vi "RT Driver VI.vi"(7 "Operation":T1, 11 "Device Reference in":T2 format="%.0x") -> (0 "Error Code":i32)   [LabVIEW 2023, in "Protection and Counter Addon Engine.lvlib"]
uses:
  Protection and Counter Addon Engine.lvlib
  <vilib>/NI VeriStand/Custom Device API/Custom Device Item Ref.ctl
  <vilib>/NI VeriStand/Custom Device API/Hardware Interface Driver VI Operation.ctl
  <vilib>/NI/NIVS Inline Async API/_VS Inline Async API/VS Inline Async API/Types/Error Handling Settings.ctl
  Addon Shared/Types/Exported.OnCompile.ctl
  Addon Shared/Types/XNET Settings.ctl
  SubModules/Frame-Protection-Support/Source/Shared/Types/Exported Frame Settings.ctl
  SubModules/Frame-Protection-Support/Source/Shared/Types/Exported Frame Type.ctl
  SubModules/Frame-Protection-Support/Source/Shared/Types/Exported Protection Settings.ctl
  SubModules/Frame-Protection-Support/Source/Shared/Types/Protection Type.ctl
  SubModules/Frame-Protection-Support/Source/Shared/Types/XNET Signal Configuration.ctl
  SubModules/Frame-Protection-Support/Source/Shared/Types/Exported Counter Settings.ctl
  SubModules/Frame-Protection-Support/Source/Shared/Types/Exported Event Trigger Type.ctl
  Addon Shared/Types/986x.ctl
  <vilib>/NI/NIVS Inline Async API/_VS Inline Async API/VS Inline Async API/VS Inline Async API.lvclass
  Types/RT Async Engine Settings.ctl
  SubModules/Frame-Protection-Support/Source/Engine/Types/RT Frame Settings.ctl
  SubModules/Frame-Protection-Support/Source/Engine/Types/RT Protection Configuration.ctl
  SubModules/Frame-Protection-Support/Source/Engine/Types/RT Frame Incoming Values.ctl
  <vilib>/NI/NIVS Inline Async API/_VS Inline Async API/VS Inline Async API/VS Inline Async API.lvclass/VS Inline Async API.ctl
  <vilib>/NI/NIVS Inline Async API/_Data Access Engine/Data Access Engine/Data Access Engine.lvclass/Data Access Engine.ctl
  <vilib>/NI/NIVS Inline Async API/_Data Access Engine/Access Type Classes/Write/Write.lvclass/Write.ctl
  <vilib>/NI/NIVS Inline Async API/_Data Access Engine/Access Type Classes/ReadWrite/ReadWrite.lvclass/ReadWrite.ctl
  <vilib>/NI/NIVS Inline Async API/_Data Access Engine/Access Type Classes/Read/Read.lvclass/Read.ctl
  SubVIs/Bitfile.Initialize.vi
  SubModules/Frame-Protection-Support/Source/Engine/SubVIs/Initialize Protection Frames Outgoing.vi
  <vilib>/NI/NIVS Inline Async API/_Data Access Engine/Data Access Engine/Methods/Data.Engine.Read Data from HW.vi
  <vilib>/NI/NIVS Inline Async API/_VS Inline Async API/Error Handling Process/SubVIs/Error.GetError.vi
  <vilib>/NI/NIVS Inline Async API/_Data Access Engine/Data Access Engine/Methods/Data.Engine.Write Data to HW.vi
  SubVIs/Bitfile.Download.vi
  <vilib>/NI/NIVS Inline Async API/_Data Access Engine/Access Type Classes/ReadWrite/ReadWrite.EngineData.vi
  <vilib>/NI/NIVS Inline Async API/_Data Access Engine/Access Type Classes/Write/Write.EngineData.vi
  <vilib>/NI/NIVS Inline Async API/_Data Access Engine/Access Type Classes/Read/Read.EngineData.vi
  <vilib>/NI VeriStand/Custom Device API/NI VeriStand - Get Channel Value by Data Reference.vi
  <vilib>/NI VeriStand/Custom Device API/NI VeriStand - Set Channel Value by Data Reference.vi
  <vilib>/NI VeriStand/Custom Device API/NI VeriStand - Get Channel Values by Block Data Reference.vi
  Addon Shared/SubVIs/GUID Lookup.vi
  <vilib>/NI VeriStand/Custom Device API/Get Item Property (Variant).vi
  <vilib>/Utility/libraryn.llb/Check if File or Folder Exists.vi
  <vilib>/Utility/error.llb/Error Cluster From Error Code.vi
  <vilib>/rvi/Utilities/XML/nirviXML_GetValue.vi
  <vilib>/rvi/Utilities/XML/nirviXML_GetValue_String.vi
  <vilib>/xnet/xnet.llb/XNET Create Session.vi
  <vilib>/xnet/xnet.llb/XNET Create Session (Frame Output Stream).vi
  <vilib>/xnet/xnet.llb/XNET Create Session (Conversion).vi
  SubModules/Frame-Protection-Support/Source/LP_CRC/Re-order Protection Configs.vi
  SubModules/Frame-Protection-Support/Source/Engine/SubVIs/Initialize Protection Frames Incoming.vi
  <vilib>/xnet/xnet.llb/XNET Create Session (Frame Input Stream).vi
  <vilib>/Utility/SystemLogging/Write to System Log.vi
  <vilib>/NI VeriStand/Custom Device API/Global Data Refs.vi
  <vilib>/NI VeriStand/Custom Device API/Custom Device API.lvlib
  Addon Shared/Protection and Counter Addon Shared.lvlib
  SubModules/Frame-Protection-Support/Source/Shared/Protection and Counter Support Shared.lvlib
  <vilib>/NI VeriStand/Custom Device Tools/Custom Device Utility Library/Custom Device Utility Library.lvlib
  SubModules/Frame-Protection-Support/Source/Engine/Protection and Counter Support Engine.lvlib
  SubModules/Frame-Protection-Support/Source/LP_CRC/LP_CRC.lvlib
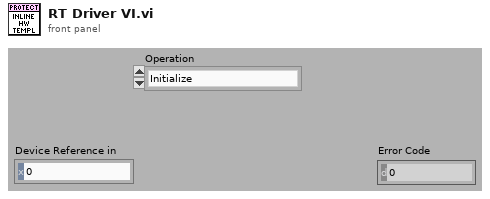
[diagram p1: front panel]
types:
  T1 = typedef "Custom Device API.lvlib/Hardware Interface Driver VI Operation.ctl" = enum16{"Initialize", "Start", "Read Data from HW", "Write Data to HW", "Close"}
  T2 = typedef "Custom Device API.lvlib/Custom Device Item Ref.ctl" = u64
  T3 = typedef "Protection and Counter Addon Engine.lvlib/RT Async Engine Settings.ctl" = cluster{"Name":string, "Priority":i32, "XNET Settings":T4, "FPGA Session":u32, "Outgoing CAN Session":refnum<k21>, "Outgoing Frame Count":i32, "Outgoing Frames":T5[], "Incoming CAN Session":refnum<k21>, "Incoming Frame Count":i32, "Incoming Frames":T5[], "Incoming Values":T12}
  T4 = typedef "Protection and Counter Addon Shared.lvlib/XNET Settings.ctl" = cluster{"Database":refnum<k21>, "Cluster":refnum<k21>, "Port":string, "Baud rate [Bd]":u64, "Termination":u32, "CAN I/O Mode":u32, "FD Baud rate [Bd]":u64, "Priority":i32, "Use Legacy":bool, "FD ISO Mode":u32}
  T5 = typedef "Protection and Counter Support Engine.lvlib/RT Frame Settings.ctl" = cluster{"Type":T6, "Frame ID":u32, "Payload Length":u32, "VS Offset":i32, "VS Length":i32, "Frame Conversion":refnum<k21>, "Frame.Data":dbl[], "Generation Period":u32, "Time Since Last Generation":u32, "Generation Iterations":u32, "Generation Counter":u32, "Has Protection?":bool, "Protection Configurations":T7[], "Has Counter?":bool, "Counter Configurations":T10[], "Has Disable?":bool, "Disable VS Index":i32, "Transmit Trigger":T11, "Trigger VS Index":i32}
  T6 = typedef "Protection and Counter Support Shared.lvlib/Exported Frame Type.ctl" = enum16{"Periodic", "Event", "Periodic/Event"}
  T7 = typedef "Protection and Counter Support Engine.lvlib/RT Protection Configuration.ctl" = cluster{"Protection Frame Index":i32, "Protection Type":T8, "Data Indeces":i32[], "Data Array":dbl[], "Check Sum Conversion":refnum<k21>, "CRC Channels":T9[], "Protection VS Index":i32, "Counter Data Index":i32, "Override Index":i32, "Override Value Index":i32, "Map":map{i32, u8[]}}
  T8 = typedef "Protection and Counter Support Shared.lvlib/Protection Type.ctl" = enum16{"Arb ID + Bytes Checksum with Inversion", "Arb ID + Bytes CRC with Inversion", "Reversed Raw Signal Checksum with Inversion", "Concatenated Two's Compliment", "LP_CRC8", "LP_Checksum", "LP_CRC8_MRS"}
  T9 = typedef "Protection and Counter Support Shared.lvlib/XNET Signal Configuration.ctl" = cluster{"Start Bit":i32, "Name":string, "Number of bits":i32, "Scale":dbl, "Offset":dbl, "Data Type":u32, "Counter":bool}
  T10 = typedef "Protection and Counter Support Shared.lvlib/Exported Counter Settings.ctl" = cluster{"Frame Index":i32, "Max Count":dbl, "VS Index":i32, "Bit Length":i64, "Override Index":i32, "Override Value Index":i32}
  T11 = typedef "Protection and Counter Support Shared.lvlib/Exported Event Trigger Type.ctl" = enum16{"Channel value change", "Trigger channel (not zero)", "Channel value change or trigger channel (not zero)", "Trigger channel (any value change)", "Channel value change or trigger channel (any value change)"}
  T12 = typedef "Protection and Counter Support Engine.lvlib/RT Frame Incoming Values.ctl" = cluster{"Signal Values":dbl[], "Signal Invalid Values":dbl[], "ProtCtr Sig Values":dbl[], "Timestamps":timestamp[], "Time Differences":dbl[], "IDs":u32[]}
  T13 = cluster{"Process":refnum<class "VS Inline Async API.lvclass">, "RT Configuration":T3}
  T14 = typedef "VS Inline Async API.lvlib/VS Inline Async API.lvclass/Error Handling Settings.ctl" = cluster{"Write to SystemLog (F)":bool}
  T15 = typedef "Protection and Counter Addon Shared.lvlib/Exported.OnCompile.ctl" = cluster{"Name":string, "XNET Settings":T4, "Frames":T16[], "986x Support":T18, "Incoming Frames":T16[]}
  T16 = typedef "Protection and Counter Support Shared.lvlib/Exported Frame Settings.ctl" = cluster{"Type":T6, "Frame ID":u32, "Payload Length":u32, "Signal XNET Paths":string[], "Frame.PrevData":dbl[], "VS Offset":i32, "VS Length":i32, "Generation Period":u32, "Has Protection?":bool, "Protection Configurations":T17[], "Has Counter":bool, "Counter Configurations":T10[], "Has Disable?":bool, "Disable VS Index":i32, "Transmit Trigger":T11, "Trigger VS Index":i32}
  T17 = typedef "Protection and Counter Support Shared.lvlib/Exported Protection Settings.ctl" = cluster{"Protection Frame Index":i32, "Protection Type":T8, "Data Indeces":i32[], "Initialized Data Array":dbl[], "Protection Signal XNET Paths":string[], "CRC Channels":T9[], "Protection VS Update Index":i32, "Override Index":i32, "Override Value Index":i32}
  T18 = typedef "Protection and Counter Addon Shared.lvlib/986x.ctl" = cluster{"Enable":bool, "RIO Device":string, "Bitfile":path}
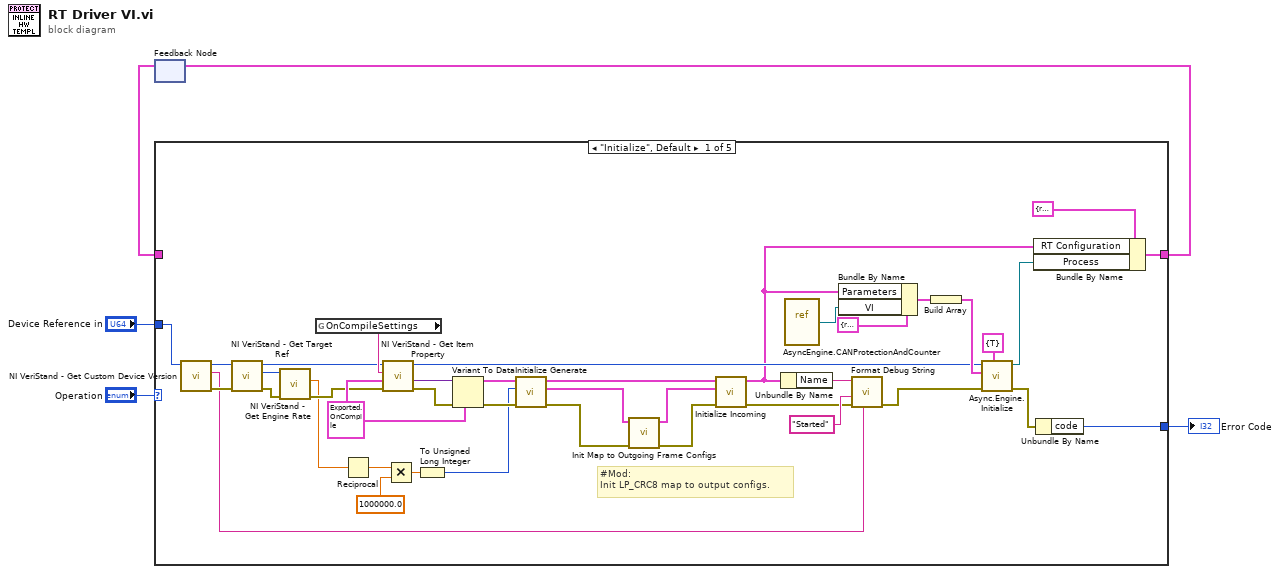
[diagram p0: block diagram]
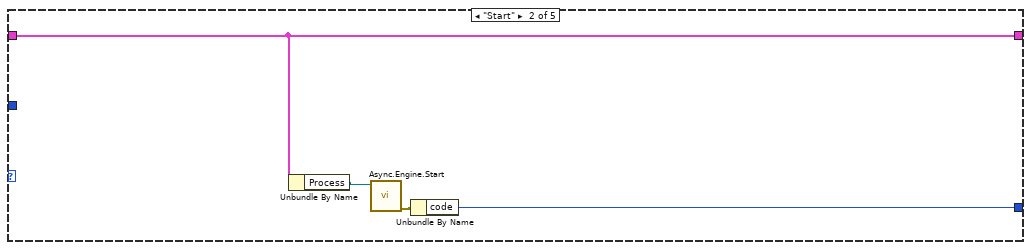
[diagram p2: hidden frame]
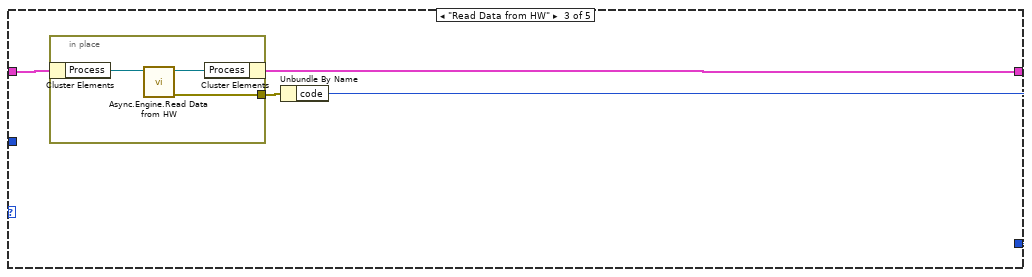
[diagram p3: hidden frame]
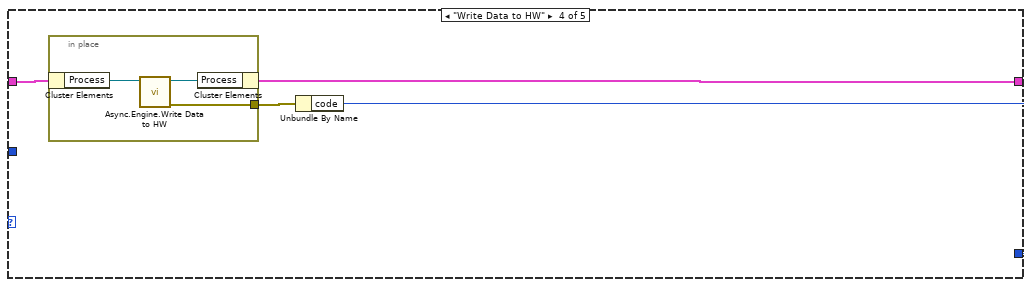
[diagram p4: hidden frame]
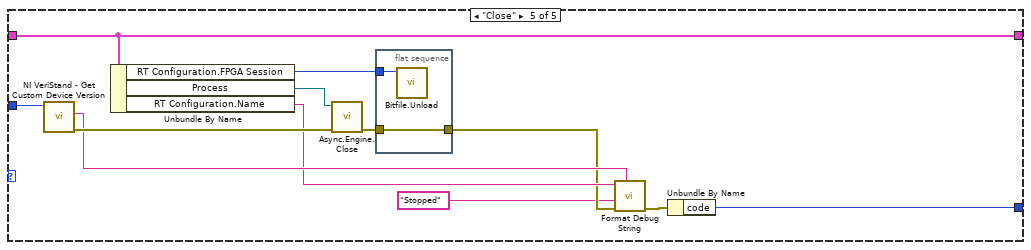
[diagram p5: hidden frame]
diagram:
  n1 = feedback #1() -> (w3:T13)  [unwired: 1 out]
  n2 = case shown="\"Initialize\", Default" "Operation" {
    tunnel: [w44 w46 w52 w60 w72] -> w4
    tunnel: w3 -> [_ w46 w53 w59 w72]
    tunnel: [w45 w49 w50 w57 w67] -> w2
    tunnel: "Device Reference in" -> [w43 _ _ _ w75]
    frame "Initialize", Default {
      w33 = T15 {"Name"="", "XNET Settings"={"Database"="", "Cluster"="", "Port"="", "Baud rate [Bd]"=500000, "Termination"=1, "CAN I/O Mode"=0, "FD Baud rate [Bd]"=500000, "Priority"=100, "Use Legacy"=FALSE, "FD ISO Mode"=0}, "Frames"=[], "986x Support"={"Enable"=FALSE, "RIO Device"="", "Bitfile"=path ""}, "Incoming Frames"=[]} ("Cluster")
      # "#Mod:\nInit LP_CRC8 map to output configs."
      n3 = call <vilib>:"NI VeriStand - Get Custom Device Version.vi"("Device Ref in"=w43) -> ("error out"=w27:errorcluster, "Value"=w16:string, "Device Ref out"=w36:T2)  [unwired: 8 in]
      n4 = call <vilib>:"NI VeriStand - Get Target Ref.vi"("error in"=w27, "Item Ref in"=w36) -> ("error out"=w26:errorcluster, "Target Ref"=w28:T2, "Item Ref out"=w29:T2)  [unwired: 6 in, 1 out]
      n5 = call <vilib>:"NI VeriStand - Get Engine Rate.vi"("error in (no error)"=w26, "Item Ref in"=w28) -> ("error out"=w25:errorcluster, "Rate (Hz)"=w24:dbl)  [unwired: 7 in, 1 out]
      n6 = global read "GUID Lookup.vi" "OnCompileSettings"() -> (w37:string)
      n7 = Reciprocal(x=w24) -> (1/x=w23:dbl)
      n8 = call-poly <vilib>:"NI VeriStand - Get Item Property.vi"("error in (no error)"=w25, "Default Value"=w33, "Property Name"=w37, "Item Ref in"=w29) -> ("error out"=w34:errorcluster, "Value"=w35:variant, "Item Ref out"=w32:T2)  [unwired: 4 in, 1 out]
      n9 = Multiply(x=w23, y=1000000.0) -> (x*y=w21:dbl)
      n10 = To Unsigned Long Integer(number=w21) -> (unsigned 32bit integer=w20:u32)
      n11 = Variant To Data(error in=w34, type=w33, Variant=w35) -> (data=w13:T15, error out=w31:errorcluster)
      n12 = call "Initialize Generate.vi"("error in (no error)"=w31, "PCL (usec)"=w20, "OnCompile Variables"=w13) -> ("error out"=w9:errorcluster, "RT Configuration"=w8:T3, "OnCompile Variables out"=w10:T15)  [unwired: 6 in]
      n13 = call "Init Map to Outgoing Frame Configs.vi"("error in (no error)"=w9, "RT Configuration In"=w8) -> ("error out"=w6:errorcluster, "RT Configuration Out"=w7:T3)  [unwired: 6 in, 1 out]
      n14 = call "Initialize Incoming.vi"("error in (no error)"=w6, "RT Configuration In"=w7, "OnCompile Variables"=w10) -> ("error out"=w12:errorcluster, "RT Configuration Out"=w11:T3)  [unwired: 7 in]
      n15 = Unbundle By Name(w11) -> ("Name"=w18:string)
      n16 = vi-ref "AsyncEngine.CANProtectionAndCounter.vi"() -> (w30:refnum<vi>)
      n17 = Bundle By Name(cluster=cluster{"VI":refnum<vi>, "Parameters":variant} {"VI"=refnum, "Parameters"=variant} ("Process"), "Parameters"=w11, "VI"=w30) -> (w40:cluster{"VI":refnum<vi>, "Parameters":variant})
      n18 = call "Format Debug String.vi"("Version"=w16, "error in (no error)"=w12, "State"="Started", "Name"=w18) -> ("error out"=w14:errorcluster)  [unwired: 7 in]
      n19 = Build Array(w40) -> (w39:cluster{"VI":refnum<vi>, "Parameters":variant}[])
      n20 = call <vilib>:"Async.Engine.Initialize.vi"("Error Log Settings"=T14 {"Write to SystemLog (F)"=TRUE}, "error in (no error)"=w14, "Processes"=w39, "Custom Device Ref"=w32) -> ("error out"=w15:errorcluster, "Async"=w42:refnum<class "VS Inline Async API.lvclass">)  [unwired: 6 in]
      n21 = Bundle By Name(cluster=T13 {"Process"=refnum, "RT Configuration"={"Name"="", "Priority"=100, "XNET Settings"={"Database"="", "Cluster"="", "Port"="", "Baud rate [Bd]"=0, "Termination"=0, "CAN I/O Mode"=0, "FD Baud rate [Bd]"=500000, "Priority"=100, "Use Legacy"=FALSE, "FD ISO Mode"=0}, "FPGA Session"=0, "Outgoing CAN Session"="", "Outgoing Frame Count"=0, "Outgoing Frames"=[], "Incoming CAN Session"="", "Incoming Frame Count"=0, "Incoming Frames"=[], "Incoming Values"={"Signal Values"=[], "Signal Invalid Values"=[], "ProtCtr Sig Values"=[], "Timestamps"=[], "Time Differences"=[], "IDs"=[]}}} ("input cluster"), "RT Configuration"=w11, "Process"=w42) -> (w44:T13)
      n22 = Unbundle By Name(w15) -> ("code"=w45:i32)
    }
    frame "Start" {
      n23 = Unbundle By Name(w46) -> ("Process"=w48:refnum<class "VS Inline Async API.lvclass">)
      n24 = call <vilib>:"Async.Engine.Start.vi"("VS Inline Async API in"=w48) -> ("error out"=w47:errorcluster)  [unwired: 9 in, 1 out]
      n25 = Unbundle By Name(w47) -> ("code"=w49:i32)
    }
    frame "Read Data from HW" {
      n26 = in-place {
        in-place-border: [w54] -> w51
        n27 = in-place-cluster #2(w53) -> ("Process"=w56:refnum<class "VS Inline Async API.lvclass">)
        n28 = call <vilib>:"Async.Engine.Read Data from HW.vi"("Async in"=w56) -> ("error out"=w54:errorcluster, "Async out"=w55:refnum<class "VS Inline Async API.lvclass">)  [unwired: 9 in]
        n29 = in-place-cluster #2("Process"=w55) -> (w52:T13)
      }
      n30 = Unbundle By Name(w51) -> ("code"=w50:i32)
    }
    frame "Write Data to HW" {
      n31 = in-place {
        in-place-border: [w61] -> w58
        n32 = in-place-cluster #3(w59) -> ("Process"=w63:refnum<class "VS Inline Async API.lvclass">)
        n33 = call <vilib>:"Async.Engine.Write Data to HW.vi"("VS Inline Async API in"=w63) -> ("error out"=w61:errorcluster, "VS Inline Async API out"=w62:refnum<class "VS Inline Async API.lvclass">)  [unwired: 9 in]
        n34 = in-place-cluster #3("Process"=w62) -> (w60:T13)
      }
      n35 = Unbundle By Name(w58) -> ("code"=w57:i32)
    }
    frame "Close" {
      n36 = call <vilib>:"NI VeriStand - Get Custom Device Version.vi"("Device Ref in"=w75) -> ("error out"=w71:errorcluster, "Value"=w70:string)  [unwired: 8 in, 1 out]
      n37 = Unbundle By Name(w72) -> ("RT Configuration.FPGA Session"=w73:u32, "Process"=w74:refnum<class "VS Inline Async API.lvclass">, "RT Configuration.Name"=w69:string)
      n38 = call <vilib>:"Async.Engine.Close.vi"("error in (no error)"=w71, "Async in"=w74) -> ("error out"=w64:errorcluster)  [unwired: 8 in, 1 out]
      n39 = flat-sequence {
        tunnel: w73 -> [w77]
        tunnel: w64 -> [w76]
        tunnel: [w76] -> w68
        frame #0 {
          n40 = call "Bitfile.Unload.vi"("Session"=w77) -> ()  [unwired: 11 in]
        }
      }
      n41 = call "Format Debug String.vi"("Version"=w70, "error in (no error)"=w68, "State"="Stopped", "Name"=w69) -> ("error out"=w65:errorcluster)  [unwired: 7 in]
      n42 = Unbundle By Name(w65) -> ("code"=w67:i32)
    }
  }
  "Error Code" <- w2
  n43 = feedback-in #1(w4) -> ()
